vi "UI sbRIO9623.vi"(8 "error in":errorcluster) -> (0 "error out":errorcluster)   [LabVIEW 2019, in "sbRIO9623.lvlib"]
uses:
  sbRIO9623.lvlib
  SubVI/IO Control.ctl
  SubVI/LED Indicator.ctl
  User Event/Controls/UE Abort Action.ctl
  <vilib>/Utility/miscctls.llb/LVPointTypeDef.ctl
  <vilib>/Utility/error.llb/Error Cluster From Error Code.vi
  <vilib>/FPGAPlugInAG/sbRIO-9623/niLvFpga_Open_sbRIO-9623.vi
  <vilib>/rvi/interface/common/dynamic/niFpgaDynamicAddResources.vi
  <vilib>/FPGAPlugInAG/Dynamic/niLvFpga_Reset_Dynamic.vi
  <vilib>/FPGAPlugInAG/Dynamic/niLvFpga_Run_Dynamic.vi
  <vilib>/rvi/errors/niLvFpgaAdjustHostInterfaceError.vi
  <vilib>/rvi/interface/common/niFpgaWaitOnOcc.vi
  <vilib>/FPGAPlugInAG/Dynamic/niLvFpga_Close_Dynamic.vi
  <vilib>/ErrorRing/Error Ring.xnode
  <vilib>/rvi/interface/nirviOpenFPGA/nirviOpenFPGA.xnode
  SubVI/LabDevice_FPGATarget_FPGA0505A2015_bllO38D53-U.lvbitx
  <vilib>/rvi/interface/nirviMethod/nirviMethod.xnode
  <vilib>/rvi/interface/nirviReadWriteControl/nirviReadWriteControl.xnode
  <vilib>/rvi/interface/nirviCloseFPGA/nirviCloseFPGA.xnode
  Queues/Queues.lvlib
  NiFpgaLv.dll
  <vilib>/rvi/interface/Simulation/niFpgaSimulationCallBeginRW.vi
  <vilib>/FPGAPlugInAG/Dynamic/niLvFpga_ConfigureFifo_Dynamic.vi
  <vilib>/rvi/errors/niLvFpgaMergeErrorWithErrorCode.vi
panel:
  in  "LED Indicator":T1
  out "Sensor Indicator":T2
  out "SiPM 2":dbl(graph) caption="Waveform Chart - dark"
  out "SiPM 1":dbl(graph) caption="Waveform Chart - dark"
  in  "I/O Control":T3
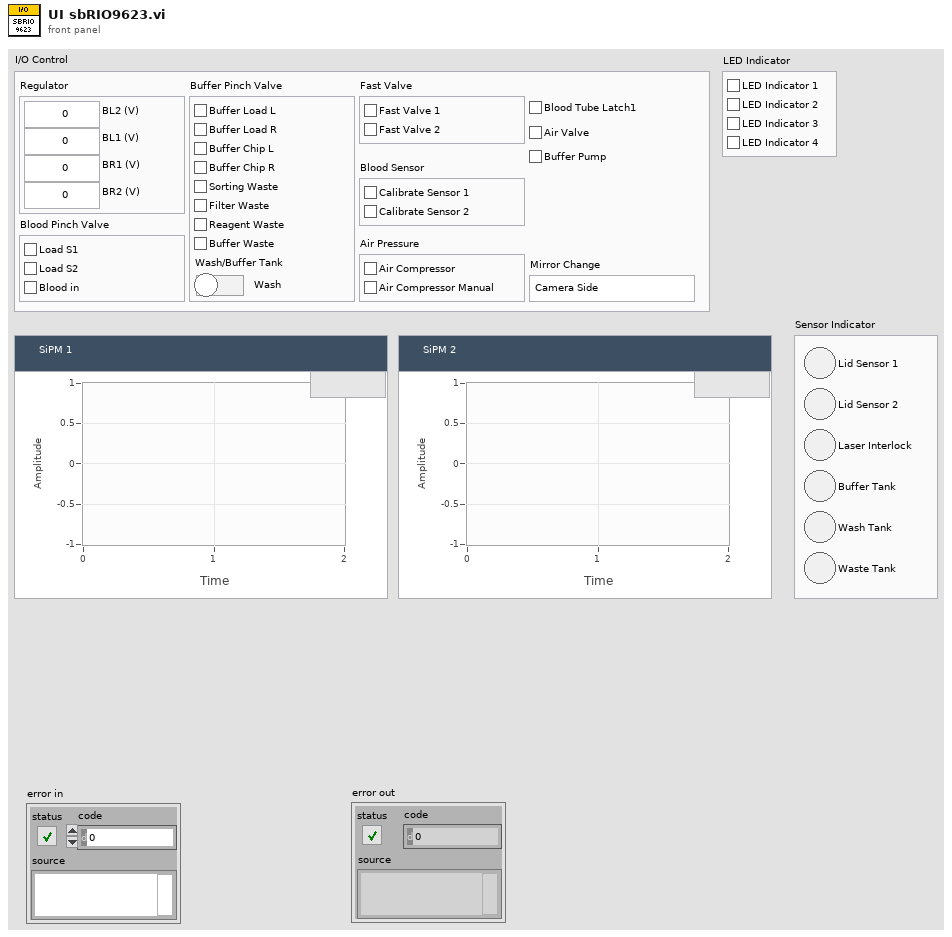
[diagram p1: front panel]
types:
  T1 = typedef "sbRIO9623.lvlib/LED Indicator.ctl" = cluster{"LED Indicator 1":bool, "LED Indicator 2":bool, "LED Indicator 3":bool, "LED Indicator 4":bool}
  T2 = cluster{"Lid Sensor 1":bool, "Lid Sensor 2":bool, "Laser Interlock":bool, "Buffer Tank":bool, "Wash Tank":bool, "Waste Tank":bool}
  T3 = typedef "sbRIO9623.lvlib/IO Control.ctl" = cluster{"Regulator":cluster{"BL2 (V)":fxp<+,16,3>, "BL1 (V)":fxp<+,16,3>, "BR1 (V)":fxp<+,16,3>, "BR2 (V)":fxp<+,16,3>}, "Buffer Pinch Valve":cluster{"Buffer Load L":bool, "Buffer Load R":bool, "Buffer Chip L":bool, "Buffer Chip R":bool, "Sorting Waste":bool, "Filter Waste":bool, "Reagent Waste":bool, "Buffer Waste":bool, "Wash/Buffer Tank":bool}, "Blood Pinch Valve":cluster{"Load S1":bool, "Load S2":bool, "Blood in":bool}, "Fast Valve":cluster{"Fast Valve 1":bool, "Fast Valve 2":bool}, "Blood Sensor":cluster{"Calibrate Sensor 1":bool, "Calibrate Sensor 2":bool}, "Air Pressure":cluster{"Air Compressor":bool, "Air Compressor Manual":bool}, "Blood Tube Latch1":bool, "Air Valve":bool, "Buffer Pump":bool, "Mirror Change":enum16{"Camera Side", "SiPM Side"}}
  T4 = cluster{"FPGA Ref":refnum<k20>, "Initialize Sucess?":bool, "Mirror Change":enum16{"Camera Side", "SiPM Side"}, "Air Pressure Control":cluster{"Air Compressor":bool, "Air Compressor (Manual)":bool, "Air Cmpressor Auto":bool}}
  T5 = typedef "UE Abort Action.ctl" = enum16{"Create", "Get", "Destroy"}
  T6 = cluster{"Wash Buffer Tank":bool, "Buffer Load L":bool, "Buffer Pump":bool}
  T7 = cluster{"Wash Buffer Tank":bool, "Buffer Load R":bool, "Buffer Pump":bool}
  T8 = cluster{"BR1":fxp<+,16,3>, "Buffer Chip R":bool, "Fast Valve 1":bool}
  T9 = cluster{"BR2":fxp<+,16,3>, "Buffer Chip R":bool, "Fast Valve 2":bool}
  T10 = typedef "LVPointTypeDef.ctl" = cluster{"Horizontal":i16, "Vertical":i16}
  T11 = typedef "sbRIO9623.lvlib/SEQ Data.ctl" = cluster{"Lid Sensor 1":bool, "Lid Sensor 2":bool, "Laser Interlock":bool, "Buffer Tank":bool, "Wash Tank":bool, "Waste Tank":bool, "SiPM 1":fxp<+,20,5>, "SiPM 2":fxp<+,20,5>, "Initialize Success?":bool, "VI Refnum":refnum<vi>}
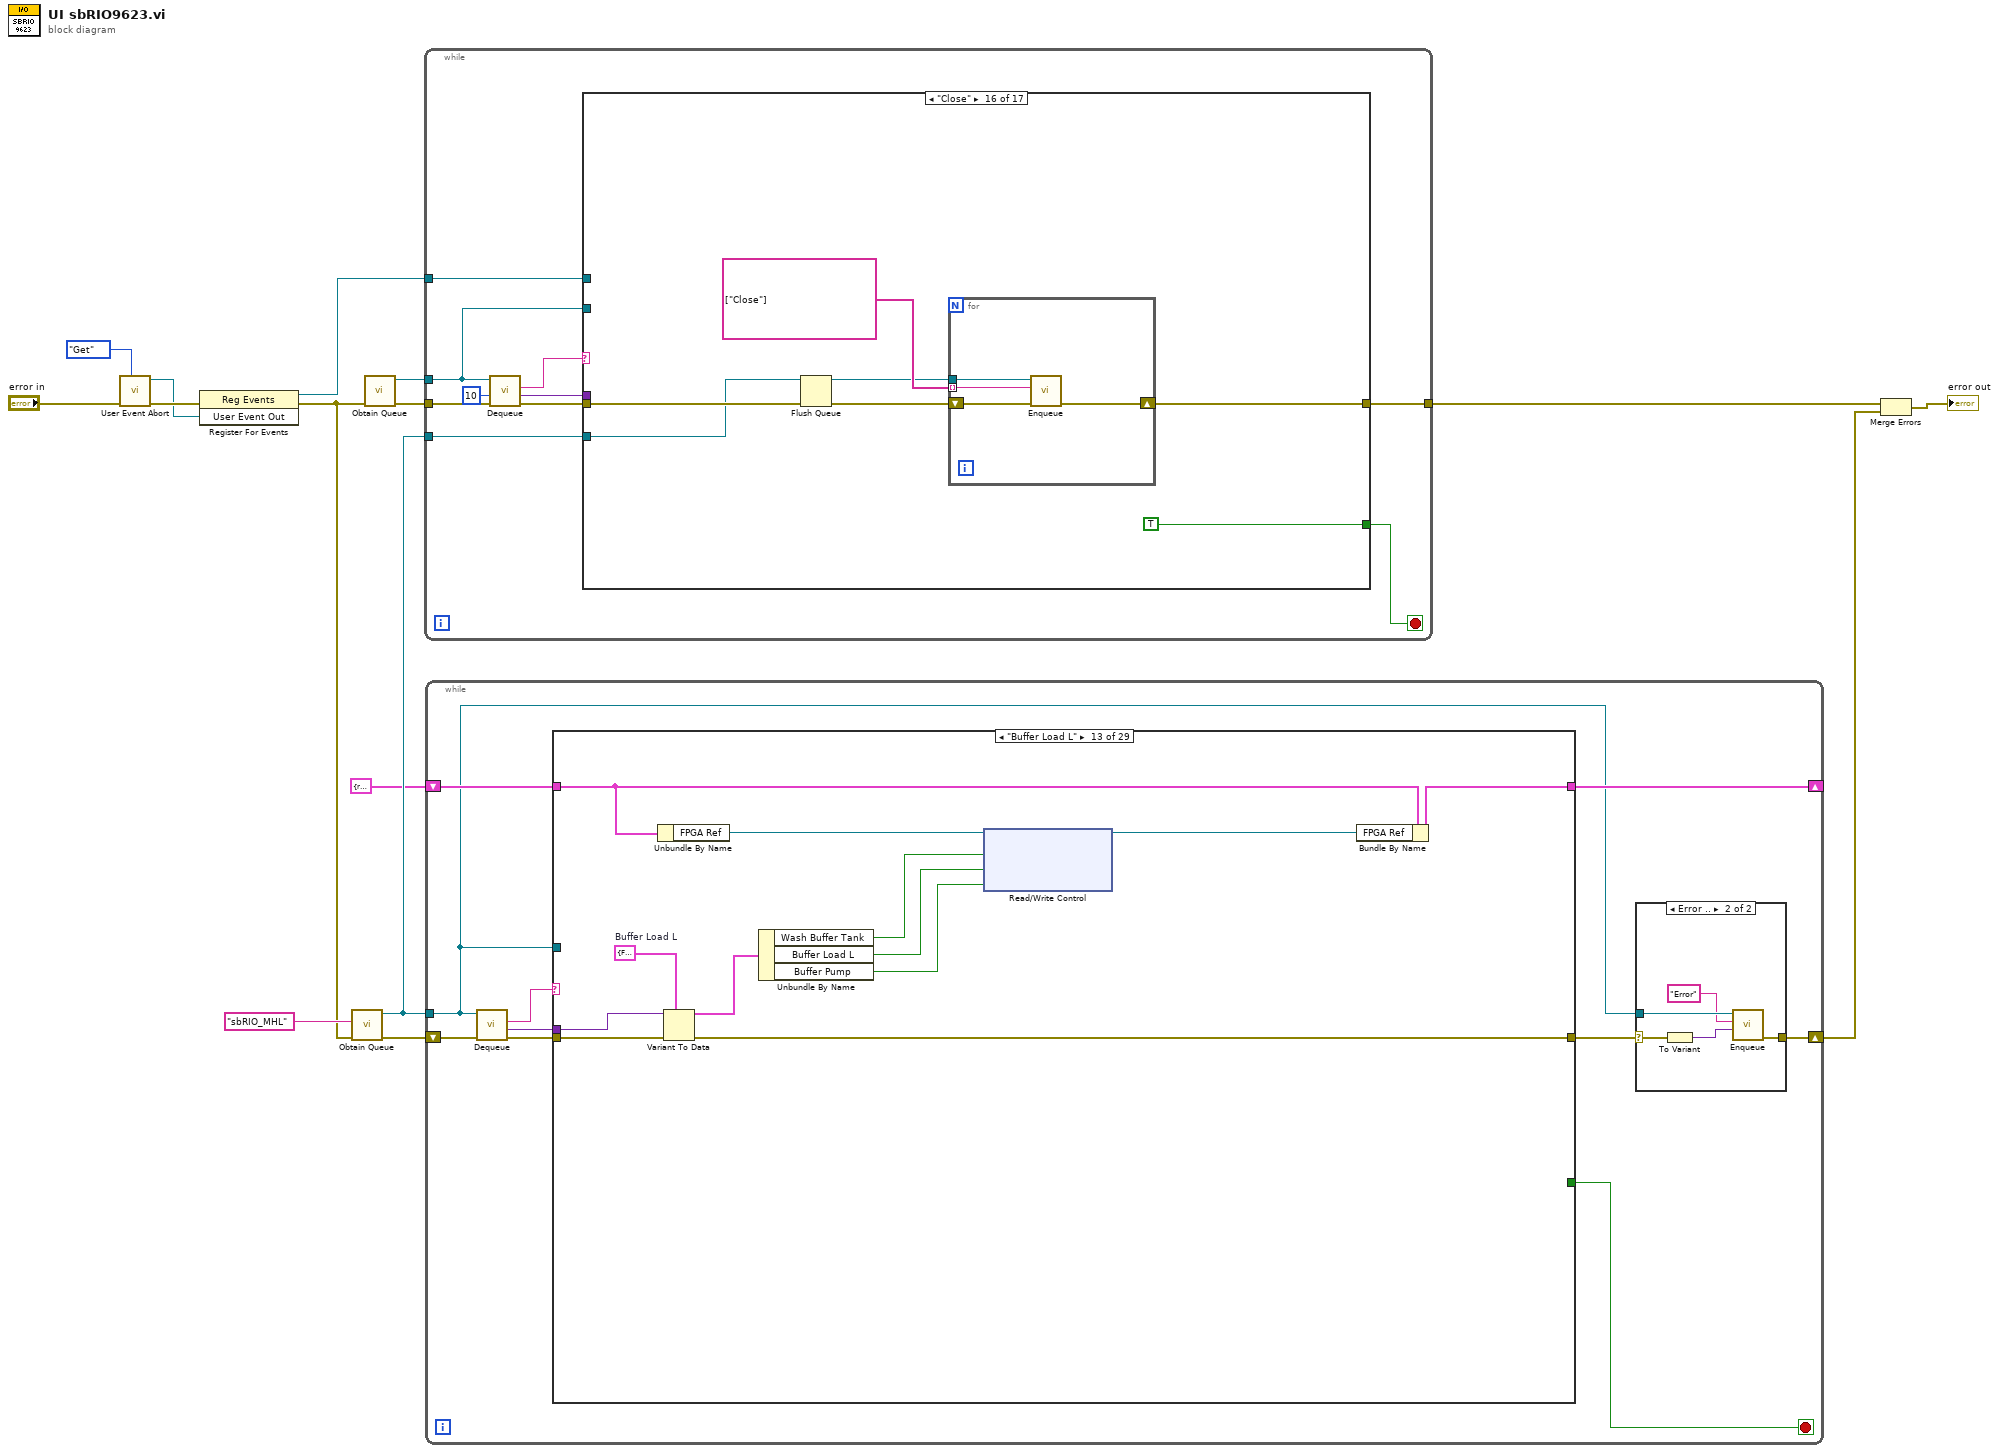
[diagram p0: block diagram]
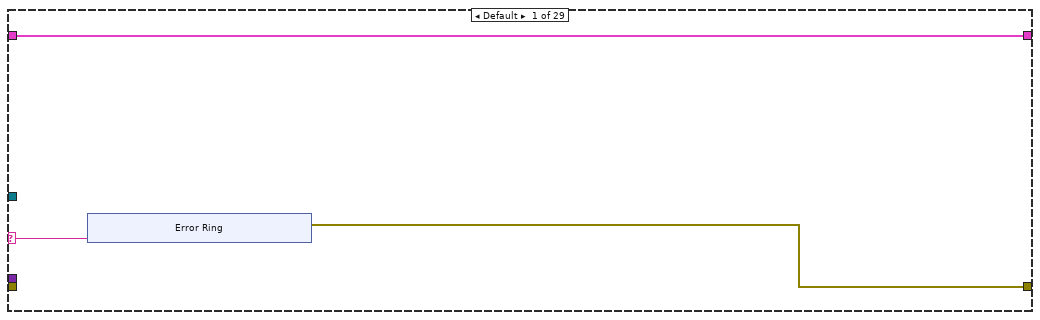
[diagram p2: hidden frame]
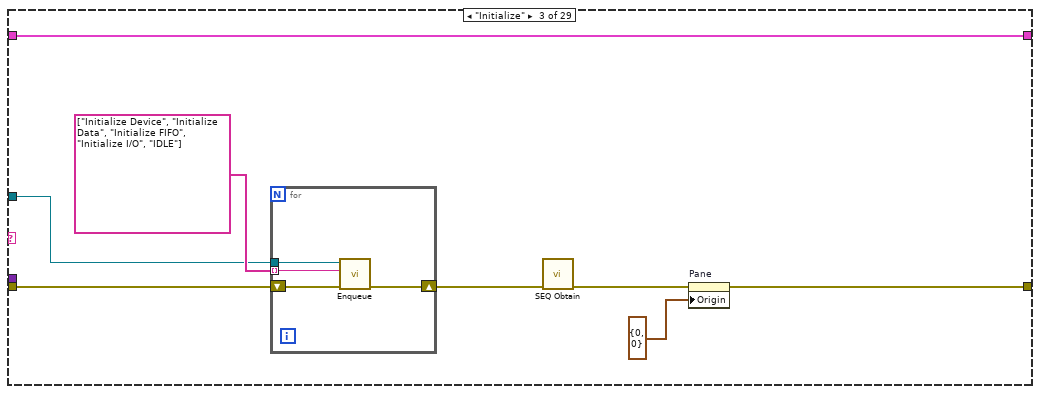
[diagram p4: hidden frame]
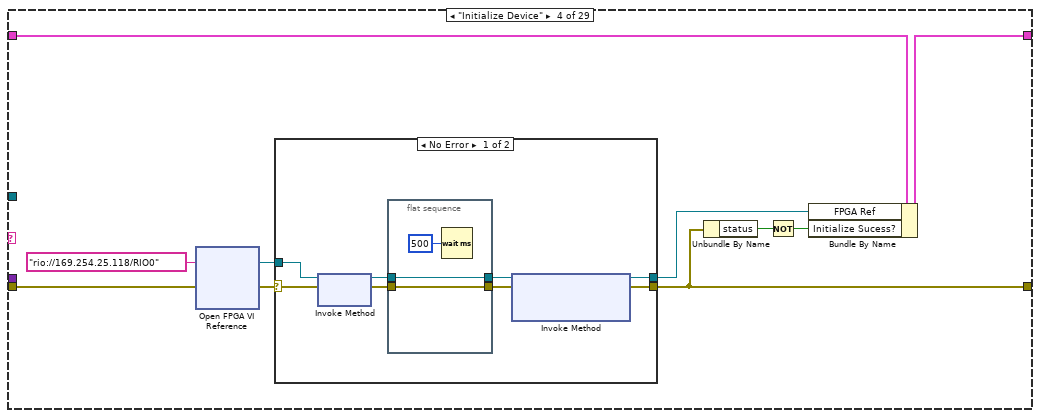
[diagram p5: hidden frame]
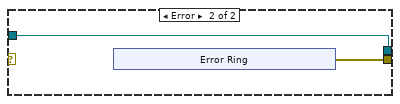
[diagram p6: hidden frame]
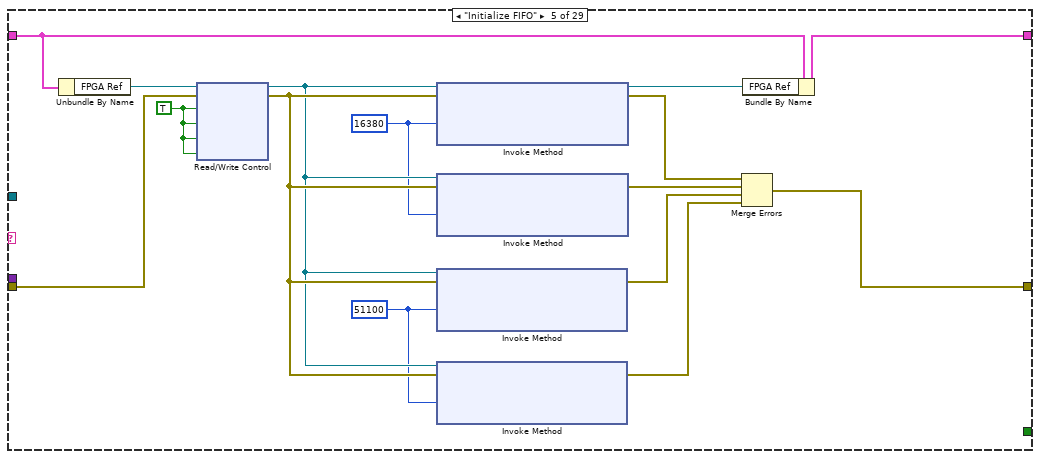
[diagram p7: hidden frame]
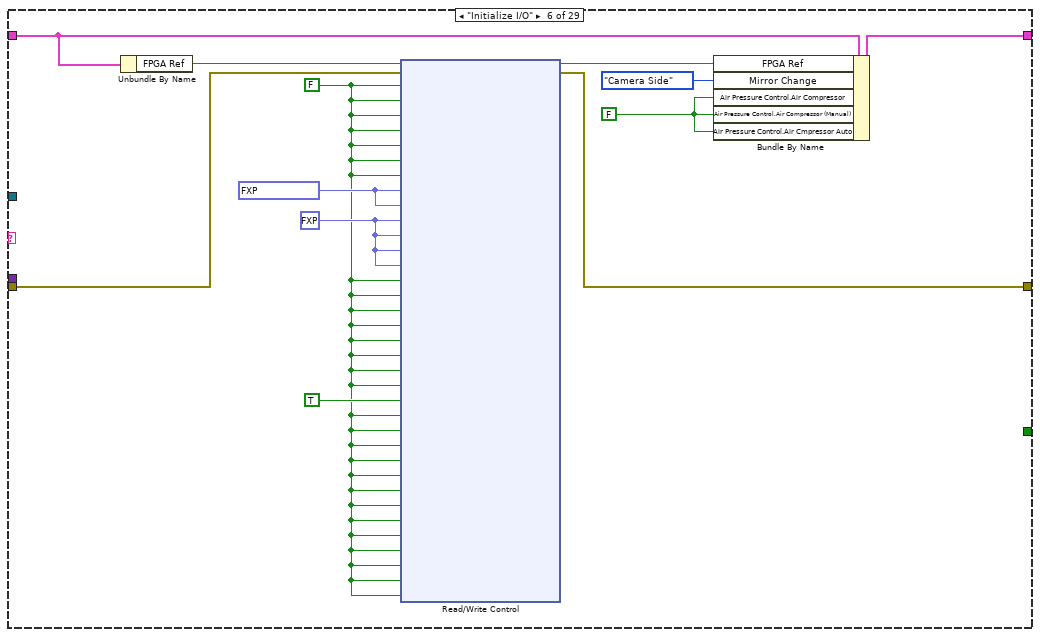
[diagram p8: hidden frame]
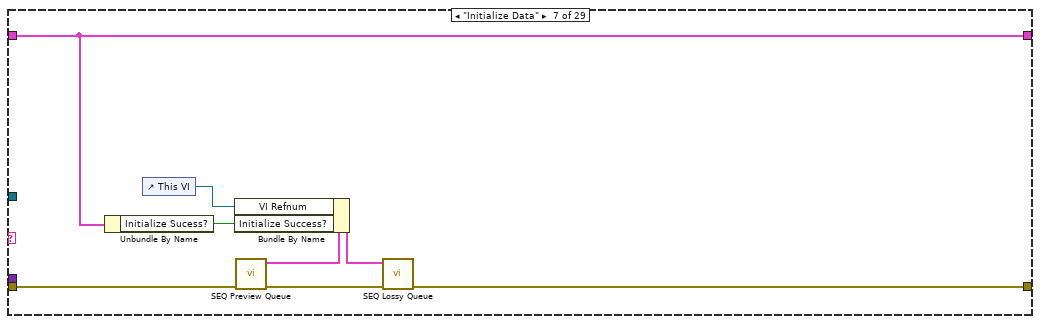
[diagram p9: hidden frame]
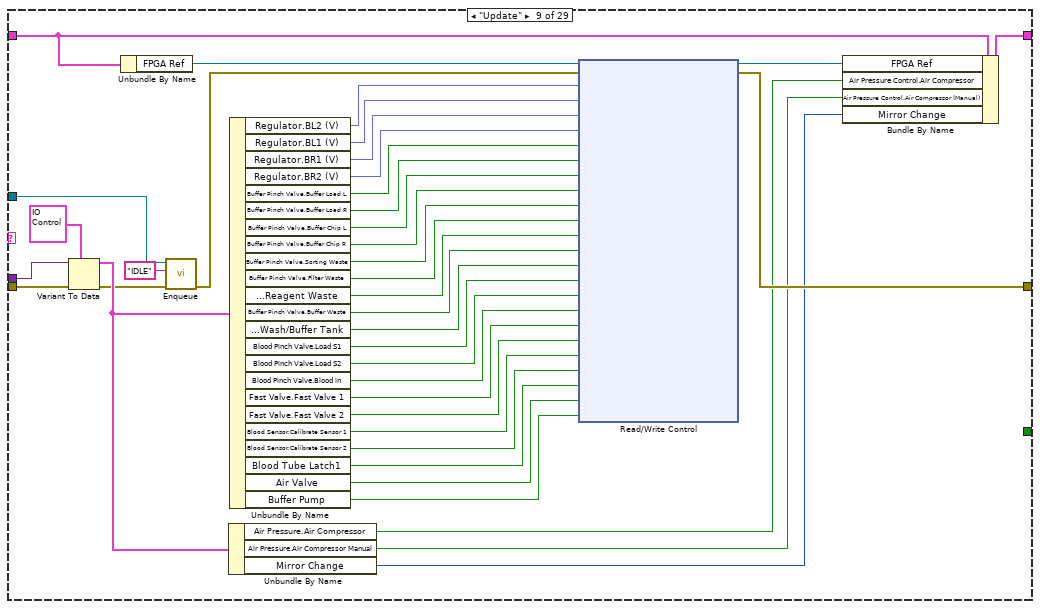
[diagram p11: hidden frame]
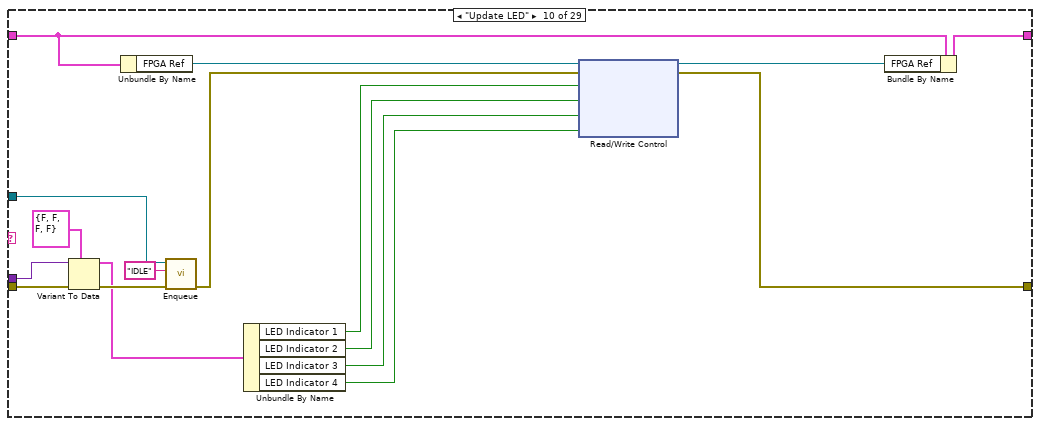
[diagram p12: hidden frame]
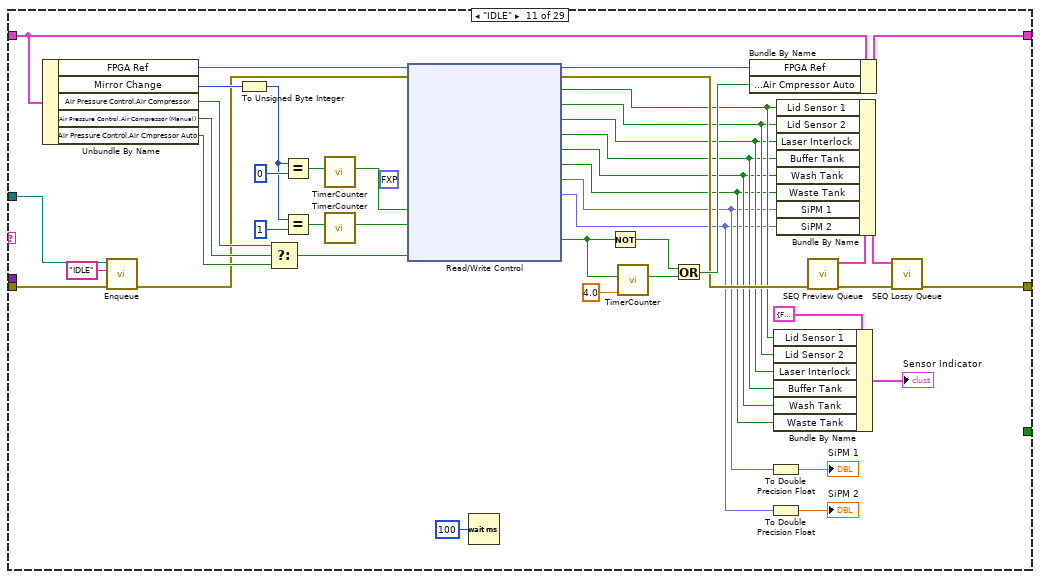
[diagram p13: hidden frame]
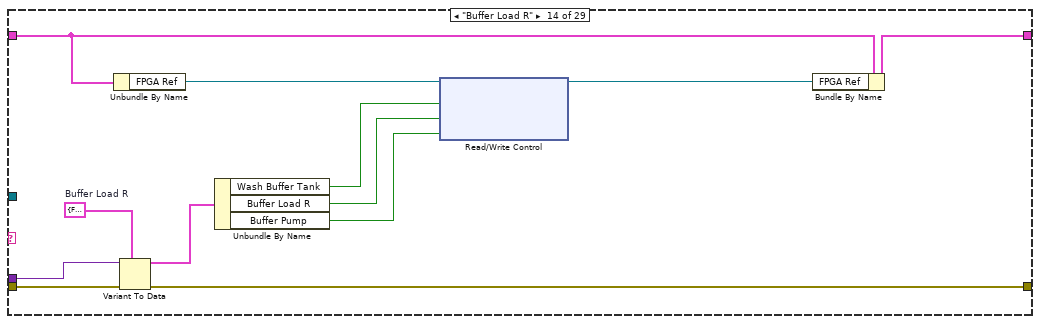
[diagram p15: hidden frame]
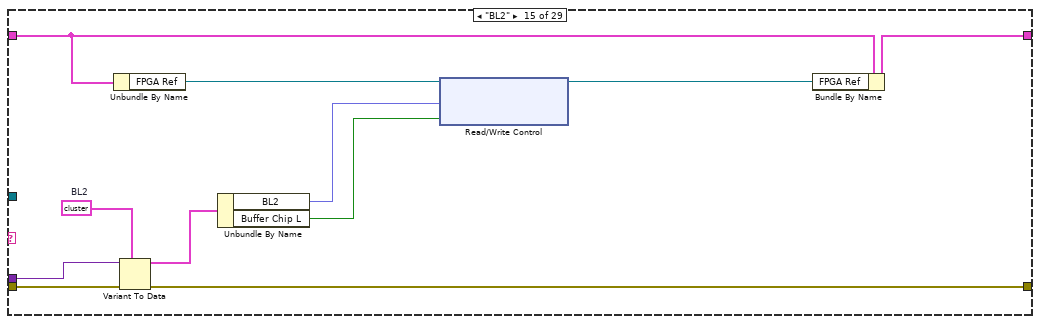
[diagram p16: hidden frame]
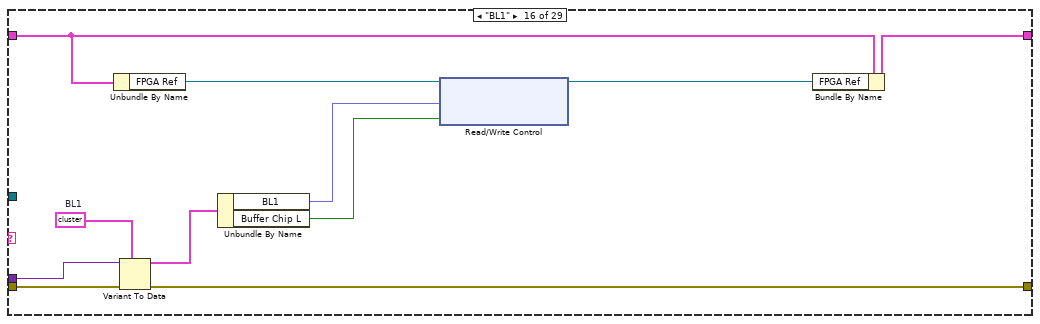
[diagram p17: hidden frame]
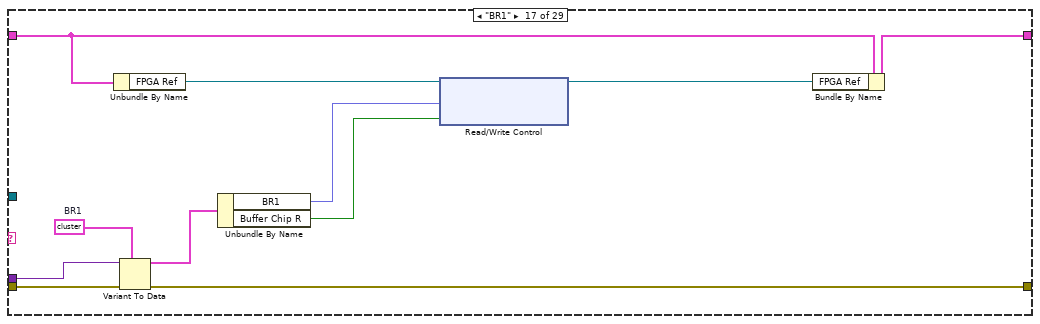
[diagram p18: hidden frame]
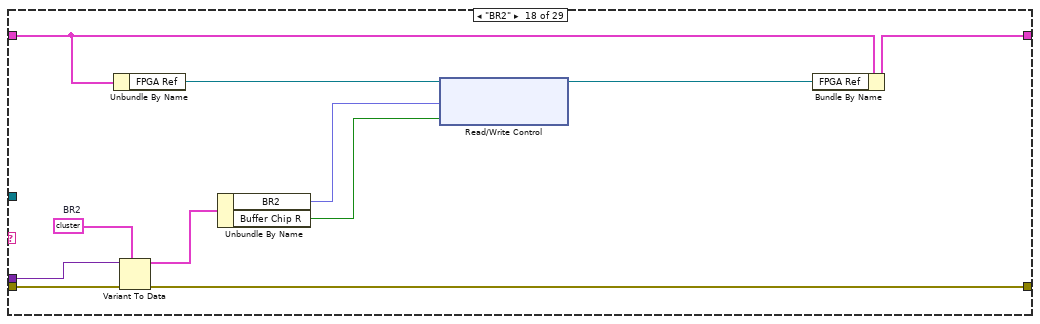
[diagram p19: hidden frame]
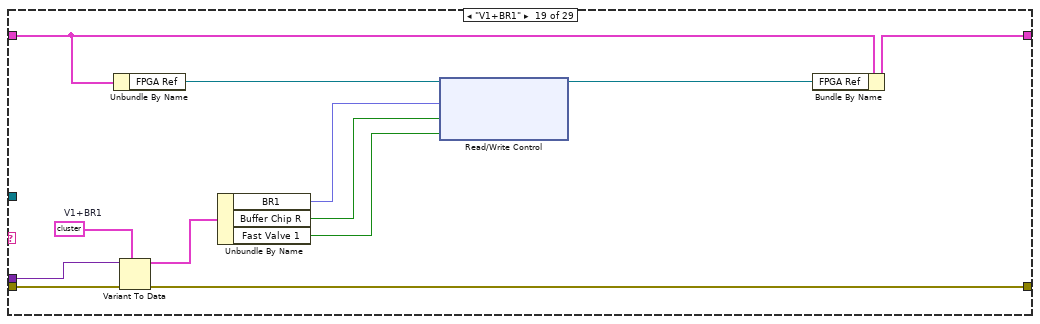
[diagram p20: hidden frame]
diagram:
  n1 = call "User Event Abort.vi"("Action"=UE_Abort_Action."Get", "Error In"="error in") -> ("Error Out"=w13:errorcluster, "User Event Out"=w12:refnum<user-event>)  [unwired: 8 in]
  n2 = register-events(error in=w13, w12) -> (reference out=w11:refnum<event-registration>, error out=w3:errorcluster)  [unwired: 1 in]
  n3 = call "Obtain Queue.vi"("Error In"=w3, "Queue Name"="sbRIO_MHL") -> ("Error Out"=w9:errorcluster, "queue out"=w5:refnum<queue>)  [unwired: 8 in]
  n4 = call "Obtain Queue.vi"("Error In"=w3) -> ("Error Out"=w2:errorcluster, "Queue out"=w1:refnum<queue>)  [unwired: 9 in]
  n5 = while {
    tunnel: w2 -> [w25]
    tunnel: w1 -> [w20]
    tunnel: [w19] -> w8
    tunnel: w11 -> [w18]
    tunnel: w5 -> [w16]
    stop <- w17 stop-if-true
    n6 = call "Dequeue.vi"("Error In"=w25, "timeout in ms (-1)"=10, "Queue in"=w20) -> ("Error Out"=w24:errorcluster, "Data"=w22:variant, "State"=w23:string)  [unwired: 5 in, 1 out]
    n7 = case shown="\"Close\"" w23 {
      selector: w23 -> [w26 _ _ _ _ _ _ _ _ _ _ _ _ _ _ _ _]
      tunnel: w24 -> [w29 w33 w46 w57 w67 w79 w91 w103 w115 w127 w139 w151 w163 w175 w187 w195 w206]
      tunnel: w22 -> [_ _ w45 w56 w66 w78 w90 w102 w114 w126 w138 w150 w162 w174 w186 _ _]
      tunnel: w20 -> [_ _ _ _ _ _ _ _ _ _ _ _ _ _ _ _ _]
      tunnel: [w29 w32 w42 w54 w65 w77 w89 w101 w113 w125 w137 w149 w161 w173 w185 w197 w205] -> w19
      tunnel: w18 -> [_ _ _ _ _ _ _ _ _ _ _ _ _ _ _ _ w204]
      tunnel: [_ _ _ _ _ _ _ _ _ _ _ _ _ _ _ TRUE _] -> w17
      tunnel: w16 -> [_ w31 w39 w50 w63 w75 w87 w99 w111 w123 w135 w147 w159 w171 w183 w192 w203]
      frame "Typo", Default {
        n8 = Concatenate Strings("Typo: " ("string"), w26) -> (w28:string)
        n9 = One Button Dialog(message=w28) -> ()  [unwired: 1 in, 1 out]
      }
      frame "Initialize" {
        n10 = for {
          tunnel: w31 -> [w35]
          shift-right: [w36] -> w32
          shift-left: w33 -> [w37]
          tunnel: string[] ["Initialize"] -> [w34] mode=indexing
          n11 = call "Enqueue.vi"("Error In"=w37, "State"=w34, "Queue in"=w35) -> ("Error Out"=w36:errorcluster)  [unwired: 7 in, 1 out]
        }
      }
      frame "Update" {
        n12 = Variant To Data(error in=w46, type=T3 {"Regulator"={"BL2 (V)"=0.0, "BL1 (V)"=0.0, "BR1 (V)"=0.0, "BR2 (V)"=0.0}, "Buffer Pinch Valve"={"Buffer Load L"=FALSE, "Buffer Load R"=FALSE, "Buffer Chip L"=FALSE, "Buffer Chip R"=FALSE, "Sorting Waste"=FALSE, "Filter Waste"=FALSE, "Reagent Waste"=FALSE, "Buffer Waste"=FALSE, "Wash/Buffer Tank"=FALSE}, "Blood Pinch Valve"={"Load S1"=FALSE, "Load S2"=FALSE, "Blood in"=FALSE}, "Fast Valve"={"Fast Valve 1"=FALSE, "Fast Valve 2"=FALSE}, "Blood Sensor"={"Calibrate Sensor 1"=FALSE, "Calibrate Sensor 2"=FALSE}, "Air Pressure"={"Air Compressor"=FALSE, "Air Compressor Manual"=FALSE}, "Blood Tube Latch1"=FALSE, "Air Valve"=FALSE, "Buffer Pump"=FALSE, "Mirror Change"=enum."Camera Side"} ("I/O Control"), Variant=w45) -> (data=w43:T3, error out=w41:errorcluster)
        n13 = To Variant(anything=w43) -> (Variant=w48:variant)
        n14 = Flush Queue(queue=w39, error in (no error)=w41) -> (queue out=w38:refnum<queue>, error out=w40:errorcluster)  [unwired: 1 out]
        n15 = call "Enqueue.vi"("Error In"=w40, "Data"=w48, "State"="Update", "Queue in"=w38) -> ("Error Out"=w42:errorcluster)  [unwired: 6 in, 1 out]
      }
      frame "Update LED" {
        n16 = Variant To Data(error in=w57, type=T1 {"LED Indicator 1"=FALSE, "LED Indicator 2"=FALSE, "LED Indicator 3"=FALSE, "LED Indicator 4"=FALSE} ("LED Indicator"), Variant=w56) -> (data=w55:T1, error out=w52:errorcluster)
        n17 = To Variant(anything=w55) -> (Variant=w59:variant)
        n18 = Flush Queue(queue=w50, error in (no error)=w52) -> (queue out=w49:refnum<queue>, error out=w51:errorcluster)  [unwired: 1 out]
        n19 = call "Enqueue.vi"("Error In"=w51, "Data"=w59, "State"="Update LED", "Queue in"=w49) -> ("Error Out"=w54:errorcluster)  [unwired: 6 in, 1 out]
      }
      frame "Buffer Load L" {
        n20 = Variant To Data(error in=w67, type=FALSE, Variant=w66) -> (data=w61:bool, error out=w62:errorcluster)
        n21 = case shown="True" w61 {
          tunnel: [w70 w71] -> w60
          frame True {
            w70 = T6 {"Wash Buffer Tank"=TRUE, "Buffer Load L"=TRUE, "Buffer Pump"=TRUE}  # Buffer Load L
          }
          frame False {
            w71 = T6 {"Wash Buffer Tank"=FALSE, "Buffer Load L"=FALSE, "Buffer Pump"=FALSE}  # Buffer Load L
          }
        }
        n22 = To Variant(anything=w60) -> (Variant=w69:variant)
        n23 = call "Enqueue.vi"("Error In"=w62, "Data"=w69, "State"="Buffer Load L", "Queue in"=w63) -> ("Error Out"=w65:errorcluster)  [unwired: 6 in, 1 out]
      }
      frame "Buffer Load R" {
        n24 = Variant To Data(error in=w79, type=FALSE, Variant=w78) -> (data=w73:bool, error out=w74:errorcluster)
        n25 = case shown="True" w73 {
          tunnel: [w82 w83] -> w72
          frame True {
            w82 = T7 {"Wash Buffer Tank"=TRUE, "Buffer Load R"=TRUE, "Buffer Pump"=TRUE}  # Buffer Load R
          }
          frame False {
            w83 = T7 {"Wash Buffer Tank"=FALSE, "Buffer Load R"=FALSE, "Buffer Pump"=FALSE}  # Buffer Load R
          }
        }
        n26 = To Variant(anything=w72) -> (Variant=w81:variant)
        n27 = call "Enqueue.vi"("Error In"=w74, "Data"=w81, "State"="Buffer Load R", "Queue in"=w75) -> ("Error Out"=w77:errorcluster)  [unwired: 6 in, 1 out]
      }
      frame "BL2" {
        n28 = Variant To Data(error in=w91, type=FALSE, Variant=w90) -> (data=w85:bool, error out=w86:errorcluster)
        n29 = case shown="True" w85 {
          tunnel: [w94 w95] -> w84
          frame True {
            w94 = cluster{"BL2":fxp<+,16,3>, "Buffer Chip L":bool} {"BL2"=0.5, "Buffer Chip L"=TRUE}  # BL2
          }
          frame False {
            w95 = cluster{"BL2":fxp<+,16,3>, "Buffer Chip L":bool} {"BL2"=0.0, "Buffer Chip L"=FALSE}  # BL2
          }
        }
        n30 = To Variant(anything=w84) -> (Variant=w93:variant)
        n31 = call "Enqueue.vi"("Error In"=w86, "Data"=w93, "State"="BL2", "Queue in"=w87) -> ("Error Out"=w89:errorcluster)  [unwired: 6 in, 1 out]
      }
      frame "BL1" {
        n32 = Variant To Data(error in=w103, type=FALSE, Variant=w102) -> (data=w97:bool, error out=w98:errorcluster)
        n33 = case shown="True" w97 {
          tunnel: [w106 w107] -> w96
          frame True {
            w106 = cluster{"BL1":fxp<+,16,3>, "Buffer Chip L":bool} {"BL1"=0.5, "Buffer Chip L"=TRUE}  # BL1
          }
          frame False {
            w107 = cluster{"BL1":fxp<+,16,3>, "Buffer Chip L":bool} {"BL1"=0.0, "Buffer Chip L"=FALSE}  # BL1
          }
        }
        n34 = To Variant(anything=w96) -> (Variant=w105:variant)
        n35 = call "Enqueue.vi"("Error In"=w98, "Data"=w105, "State"="BL1", "Queue in"=w99) -> ("Error Out"=w101:errorcluster)  [unwired: 6 in, 1 out]
      }
      frame "BR1" {
        n36 = Variant To Data(error in=w115, type=FALSE, Variant=w114) -> (data=w109:bool, error out=w110:errorcluster)
        n37 = case shown="True" w109 {
          tunnel: [w118 w119] -> w108
          frame True {
            w118 = cluster{"BR1":fxp<+,16,3>, "Buffer Chip R":bool} {"BR1"=0.5, "Buffer Chip R"=TRUE}  # BR1
          }
          frame False {
            w119 = cluster{"BR1":fxp<+,16,3>, "Buffer Chip R":bool} {"BR1"=0.0, "Buffer Chip R"=FALSE}  # BR1
          }
        }
        n38 = To Variant(anything=w108) -> (Variant=w117:variant)
        n39 = call "Enqueue.vi"("Error In"=w110, "Data"=w117, "State"="BR1", "Queue in"=w111) -> ("Error Out"=w113:errorcluster)  [unwired: 6 in, 1 out]
      }
      frame "BR2" {
        n40 = Variant To Data(error in=w127, type=FALSE, Variant=w126) -> (data=w121:bool, error out=w122:errorcluster)
        n41 = case shown="True" w121 {
          tunnel: [w130 w131] -> w120
          frame True {
            w130 = cluster{"BR2":fxp<+,16,3>, "Buffer Chip R":bool} {"BR2"=0.5, "Buffer Chip R"=TRUE}  # BR2
          }
          frame False {
            w131 = cluster{"BR2":fxp<+,16,3>, "Buffer Chip R":bool} {"BR2"=0.0, "Buffer Chip R"=FALSE}  # BR2
          }
        }
        n42 = To Variant(anything=w120) -> (Variant=w129:variant)
        n43 = call "Enqueue.vi"("Error In"=w122, "Data"=w129, "State"="BR2", "Queue in"=w123) -> ("Error Out"=w125:errorcluster)  [unwired: 6 in, 1 out]
      }
      frame "V1+BR1" {
        n44 = Variant To Data(error in=w139, type=FALSE, Variant=w138) -> (data=w133:bool, error out=w134:errorcluster)
        n45 = case shown="True" w133 {
          tunnel: [w142 w143] -> w132
          frame True {
            w142 = T8 {"BR1"=0.5, "Buffer Chip R"=TRUE, "Fast Valve 1"=TRUE}  # V1+BR1
          }
          frame False {
            w143 = T8 {"BR1"=0.0, "Buffer Chip R"=FALSE, "Fast Valve 1"=FALSE}  # V1+BR1
          }
        }
        n46 = To Variant(anything=w132) -> (Variant=w141:variant)
        n47 = call "Enqueue.vi"("Error In"=w134, "Data"=w141, "State"="V1+BR1", "Queue in"=w135) -> ("Error Out"=w137:errorcluster)  [unwired: 6 in, 1 out]
      }
      frame "V2+BR2" {
        n48 = Variant To Data(error in=w151, type=FALSE, Variant=w150) -> (data=w145:bool, error out=w146:errorcluster)
        n49 = case shown="True" w145 {
          tunnel: [w154 w155] -> w144
          frame True {
            w154 = T9 {"BR2"=0.5, "Buffer Chip R"=TRUE, "Fast Valve 2"=TRUE}  # V2+BR2
          }
          frame False {
            w155 = T9 {"BR2"=0.0, "Buffer Chip R"=FALSE, "Fast Valve 2"=FALSE}  # V2+BR2
          }
        }
        n50 = To Variant(anything=w144) -> (Variant=w153:variant)
        n51 = call "Enqueue.vi"("Error In"=w146, "Data"=w153, "State"="V2+BR2", "Queue in"=w147) -> ("Error Out"=w149:errorcluster)  [unwired: 6 in, 1 out]
      }
      frame "REA" {
        n52 = Variant To Data(error in=w163, type=FALSE, Variant=w162) -> (data=w157:bool, error out=w158:errorcluster)
        n53 = case shown="True" w157 {
          tunnel: [w166 w167] -> w156
          frame True {
            w166 = cluster{"BL2":fxp<+,16,3>, "Air Valve":bool} {"BL2"=0.5, "Air Valve"=TRUE}  # REA
          }
          frame False {
            w167 = cluster{"BL2":fxp<+,16,3>, "Air Valve":bool} {"BL2"=0.0, "Air Valve"=FALSE}  # REA
          }
        }
        n54 = To Variant(anything=w156) -> (Variant=w165:variant)
        n55 = call "Enqueue.vi"("Error In"=w158, "Data"=w165, "State"="REA", "Queue in"=w159) -> ("Error Out"=w161:errorcluster)  [unwired: 6 in, 1 out]
      }
      frame "SW1/2" {
        n56 = Variant To Data(error in=w175, type=FALSE, Variant=w174) -> (data=w169:bool, error out=w170:errorcluster)
        n57 = case shown="True" w169 {
          tunnel: [w178 w179] -> w168
          frame True {
            w178 = cluster{"Sorting Waste":bool} {"Sorting Waste"=TRUE}  # SW1/2
          }
          frame False {
            w179 = cluster{"Sorting Waste":bool} {"Sorting Waste"=FALSE}  # SW1/2
          }
        }
        n58 = To Variant(anything=w168) -> (Variant=w177:variant)
        n59 = call "Enqueue.vi"("Error In"=w170, "Data"=w177, "State"="SW1/2", "Queue in"=w171) -> ("Error Out"=w173:errorcluster)  [unwired: 6 in, 1 out]
      }
      frame "FW1/2" {
        n60 = Variant To Data(error in=w187, type=FALSE, Variant=w186) -> (data=w181:bool, error out=w182:errorcluster)
        n61 = case shown="True" w181 {
          tunnel: [w190 w191] -> w180
          frame True {
            w190 = cluster{"Filter Waste":bool} {"Filter Waste"=TRUE}  # FW1/2
          }
          frame False {
            w191 = cluster{"Filter Waste":bool} {"Filter Waste"=FALSE}  # FW1/2
          }
        }
        n62 = To Variant(anything=w180) -> (Variant=w189:variant)
        n63 = call "Enqueue.vi"("Error In"=w182, "Data"=w189, "State"="FW1/2", "Queue in"=w183) -> ("Error Out"=w185:errorcluster)  [unwired: 6 in, 1 out]
      }
      frame "Close" {
        n64 = Flush Queue(queue=w192, error in (no error)=w195) -> (queue out=w193:refnum<queue>, error out=w194:errorcluster)  [unwired: 1 out]
        n65 = for {
          tunnel: w193 -> [w200]
          shift-right: [w201] -> w197
          shift-left: w194 -> [w202]
          tunnel: string[] ["Close"] -> [w199] mode=indexing
          n66 = call "Enqueue.vi"("Error In"=w202, "State"=w199, "Queue in"=w200) -> ("Error Out"=w201:errorcluster)  [unwired: 7 in, 1 out]
        }
      }
      frame "Idle" {
        n67 = event shown="[0] Timeout" {
          selector: w204 -> [_ _ _ w218]
          dyn-events: _ -> [_ _ _ _]
          timeout: 10 -> [_ _ _ _]
          tunnel: w206 -> [w208 w211 w213 w216]
          tunnel: [w208 w210 w212 w217] -> w205
          tunnel: w203 -> [_ _ _ _]
          event Timeout {
            n68 = event-data() -> ()  [unwired: 1 in, 3 out]
          }
          event Value Change {
            n69 = event-data() -> ()  [unwired: 1 in, 6 out]
            n70 = call "Update.vi"("Error In"=w211, "I/O Control"="I/O Control") -> ("Error Out"=w210:errorcluster)  [unwired: 9 in]
          }
          event Value Change {
            n71 = event-data() -> ()  [unwired: 1 in, 6 out]
            n72 = call "Update LED.vi"("Error In"=w213, "LED Indicator"="LED Indicator") -> ("Error Out"=w212:errorcluster)  [unwired: 9 in]
          }
          event User Event {
            n73 = event-data() -> ()  [unwired: 1 in, 4 out]
            n74 = call "Close.vi"("Error In"=w216) -> ("Error Out"=w215:errorcluster)  [unwired: 10 in]
            n75 = Unregister For Events(event registration refnum=w218, error in=w215) -> (error out=w217:errorcluster)
          }
        }
      }
    }
  }
  n76 = while {
    tunnel: w5 -> [w220]
    shift-right: [w223] -> _
    shift-left: T4 {"FPGA Ref"=refnum, "Initialize Sucess?"=FALSE, "Mirror Change"=enum."Camera Side", "Air Pressure Control"={"Air Compressor"=FALSE, "Air Compressor (Manual)"=FALSE, "Air Cmpressor Auto"=FALSE}} -> [w224]
    shift-right: [w222] -> w6
    shift-left: w9 -> [w228]
    stop <- w219 stop-if-true
    n77 = call "Dequeue.vi"("Error In"=w228, "Queue in"=w220) -> ("Error Out"=w225:errorcluster, "Data"=w226:variant, "State"=w227:string)  [unwired: 6 in, 1 out]
    n78 = case shown="\"Buffer Load L\"" w227 {
      selector: w227 -> [w230 _ _ _ _ _ _ _ _ _ _ _ _ _ _ _ _ _ _ _ _ _ _ _ _ _ _ _ _]
      tunnel: w220 -> [_ _ w246 _ _ _ _ _ w319 w364 w375 _ _ _ _ _ _ _ _ _ _ _ _ _ _ _ w554 _ w568]
      tunnel: w226 -> [_ _ _ _ _ _ _ _ w353 w370 _ _ w429 w441 w452 w463 w474 w485 w497 w509 w520 w530 w540 _ w546 _ _ _ _]
      tunnel: w225 -> [_ w239 w247 w262 w293 w301 w315 w317 w354 w371 w377 w417 w430 w442 w453 w464 w475 w486 w498 w510 w521 w531 w541 w543 w547 w551 w555 w564 w569]
      tunnel: w224 -> [w231 w240 w245 w258 w295 w307 w310 w316 w356 w373 w416 w418 w428 w440 w451 w462 w473 w484 w496 w508 w519 w529 w539 w542 w544 w550 w552 w563 w567]
      tunnel: [w231 w240 w245 w257 w285 w305 w310 w316 w355 w372 w414 w418 w427 w439 w450 w461 w472 w483 w495 w507 w518 w528 w538 w542 w544 w550 w552 w563 w567] -> w223
      tunnel: [w229 w239 w242 w255 w286 w299 w313 w317 w349 w367 w392 w417 w424 w436 w446 w457 w468 w479 w491 w503 w514 w524 w534 w543 errorcluster {"status"=FALSE, "code"=0, "source"=""} ("Error Out") w551 w553 w561 w565] -> w221
      tunnel: [_ _ _ _ _ _ _ _ _ _ _ _ _ _ _ _ _ _ _ _ _ _ _ _ _ _ _ _ TRUE] -> w219
      frame Default {
        n79 = xnode "Error Ring"("parameter 0"=w230) -> ("error out"=w229:errorcluster)
      }
      frame "------Initialize------" {
      }
      frame "Initialize" {
        n80 = for {
          tunnel: w246 -> [w250]
          shift-right: [w251] -> w244
          shift-left: w247 -> [w252]
          tunnel: string[] ["Initialize Device", "Initialize Data", "Initialize FIFO", "Initialize I/O", "IDLE"] -> [w249] mode=indexing
          n81 = call "Enqueue.vi"("Error In"=w252, "State"=w249, "Queue in"=w250) -> ("Error Out"=w251:errorcluster)  [unwired: 7 in, 1 out]
        }
        n82 = call "SEQ Obtain.vi"("error in"=w244) -> ("error out"=w243:errorcluster)  [unwired: 9 in, 1 out]
        n83 = property on="Pane" class="Pane"(error in=w243, "Origin"=T10 {"Horizontal"=0, "Vertical"=0}) -> (error out=w242:errorcluster)  [unwired: 1 in, 1 out]
      }
      frame "Initialize Device" {
        n84 = xnode "Open FPGA VI Reference"("error in"=w262, "resource name"=tag "rio://169.254.25.118/RIO0") -> ("FPGA VI Reference Out"=w260:refnum<k20>, "error out"=w259:errorcluster)
        n85 = case shown="No Error" w259 {
          selector: w259 -> [w269 _]
          tunnel: w260 -> [w270 w274]
          tunnel: [w264 w275] -> w255
          tunnel: [w263 w274] -> w256
          frame No Error {
            n86 = xnode "Invoke Method"("FPGA VI Reference In"=w270, "error in"=w269) -> ("FPGA VI Reference Out"=w267:refnum<k20>, "error out"=w268:errorcluster)
            n87 = flat-sequence {
              tunnel: w268 -> [w273]
              tunnel: [w273] -> w266
              tunnel: w267 -> [w272]
              tunnel: [w272] -> w265
              frame #0 {
                n88 = Wait (ms)(milliseconds to wait=u32 500) -> ()  [unwired: 1 out]
              }
            }
            n89 = xnode "Invoke Method"("FPGA VI Reference In"=w265, "error in"=w266) -> ("FPGA VI Reference Out"=w263:refnum<k20>, "error out"=w264:errorcluster)  [unwired: 1 in]
          }
          frame Error {
            n90 = xnode "Error Ring"() -> ("error out"=w275:errorcluster)
          }
        }
        n91 = Unbundle By Name(w255) -> ("status"=w254:bool)
        n92 = Not(x=w254) -> (.not. x?=w253:bool)
        n93 = Bundle By Name(cluster=w258, "FPGA Ref"=w256, "Initialize Sucess?"=w253) -> (w257:T4)
      }
      frame "Initialize FIFO" {
        w281 = u32 16380 ("Requested Depth")
        w282 = u32 51100 ("Requested Depth")
        w292 = TRUE ("LED Fan-1")
        n94 = Unbundle By Name(w295) -> ("FPGA Ref"=w294:refnum<k20>)
        n95 = xnode "Read/Write Control"("FPGA VI Reference In"=w294, "error in"=w293, "LED Fan-1"=w292, "LED Fan-2"=w292, "LED Fan-3"=w292, "LED Fan-4"=w292) -> ("FPGA VI Reference Out"=w284:refnum<k20>, "error out"=w291:errorcluster)
        n96 = xnode "Invoke Method"("FPGA VI Reference In"=w284, "error in"=w291, "Requested Depth"=w281) -> ("FPGA VI Reference Out"=w283:refnum<k20>, "error out"=w290:errorcluster)  [unwired: 1 out]
        n97 = xnode "Invoke Method"("FPGA VI Reference In"=w284, "error in"=w291, "Requested Depth"=w281) -> ("error out"=w289:errorcluster)  [unwired: 2 out]
        n98 = xnode "Invoke Method"("FPGA VI Reference In"=w284, "error in"=w291, "Requested Depth"=w282) -> ("error out"=w288:errorcluster)  [unwired: 2 out]
        n99 = xnode "Invoke Method"("FPGA VI Reference In"=w284, "error in"=w291, "Requested Depth"=w282) -> ("error out"=w287:errorcluster)  [unwired: 2 out]
        n100 = Merge Errors(w290, w289, w288, w287) -> (w286:errorcluster)
        n101 = Bundle By Name(cluster=w295, "FPGA Ref"=w283) -> (w285:T4)
      }
      frame "Initialize I/O" {
        w296 = FALSE ("Air Pressure Control.Air Compressor (Manual)")
        w303 = fxp<+,16,3> 0.0 ("regulatorcontrol2 (V)")
        w304 = fxp<+,20,5> 31.9990234375 ("TriggerLevel_sipm1")
        w298 = FALSE ("Baseline data?")
        n102 = Unbundle By Name(w307) -> ("FPGA Ref"=w306:refnum<k20>)
        n103 = xnode "Read/Write Control"("FPGA VI Reference In"=w306, "error in"=w301, "Baseline data?"=w298, "Air Compressor"=w298, "Indicator LED-1"=w298, "Indicator LED-2"=w298, "Indicator LED-3"=w298, "Indicator LED-4"=w298, "Buzzer Alarm"=w298, "TriggerLevel_sipm1"=w304, "TriggerLevel_sipm2"=w304, "regulatorcontrol2 (V)"=w303, "regulatorcontrol1 (V)"=w303, "regulatorcontrol3 (V)"=w303, "regulatorcontrol4 (V)"=w303, "Buffer Pinch Valve- 1"=w298, "Buffer Pinch Valve- 2"=w298, "Buffer Pinch Valve- 3"=w298, "Buffer Pinch Valve- 4"=w298, "Buffer Pinch Valve- 5"=w298, "Buffer Pinch Valve- 6"=w298, "Buffer Pinch Valve- 7"=w298, "Buffer Pinch Valve- 8"=w298, "Buffer Pinch Valve- 9"=TRUE, "Auto Fast Valve1"=w298, "Auto Fast Valve2"=w298, "FastValve1"=w298, "FastValve2"=w298, "Air Valve"=w298, "Blood Tube Latch-A"=w298, "Blood Tube Latch-B"=w298, "Buffer Pump"=w298, "Blood Sensor Calibration-1"=w298, "Blood Sensor Calibration-2"=w298, "Blood Pinch Valve-1"=w298, "Blood Pinch Valve-2"=w298, "Blood Pinch Valve-3"=w298) -> ("FPGA VI Reference Out"=w300:refnum<k20>, "error out"=w299:errorcluster)
        n104 = Bundle By Name(cluster=w307, "FPGA Ref"=w300, "Mirror Change"=enum16{"Camera Side", "SiPM Side"}."Camera Side", "Air Pressure Control.Air Compressor"=w296, "Air Pressure Control.Air Compressor (Manual)"=w296, "Air Pressure Control.Air Cmpressor Auto"=w296) -> (w305:T4)
      }
      frame "Initialize Data" {
        n105 = Unbundle By Name(w310) -> ("Initialize Sucess?"=w309:bool)
        n106 = control-ref of="This VI"() -> (w308:refnum<vi>)
        n107 = call "SEQ Preview Queue.vi"("error in"=w315) -> ("error out"=w314:errorcluster, "SEQ Data"=w312:T11)  [unwired: 9 in]
        n108 = Bundle By Name(cluster=w312, "VI Refnum"=w308, "Initialize Success?"=w309) -> (w311:T11)
        n109 = call "SEQ Lossy Queue.vi"("error in"=w314, "SEQ Data"=w311) -> ("error out"=w313:errorcluster)  [unwired: 9 in]
      }
      frame "------Functions------" {
      }
      frame "Update" {
        n110 = Variant To Data(error in=w354, type=T3 {"Regulator"={"BL2 (V)"=0.0, "BL1 (V)"=0.0, "BR1 (V)"=0.0, "BR2 (V)"=0.0}, "Buffer Pinch Valve"={"Buffer Load L"=FALSE, "Buffer Load R"=FALSE, "Buffer Chip L"=FALSE, "Buffer Chip R"=FALSE, "Sorting Waste"=FALSE, "Filter Waste"=FALSE, "Reagent Waste"=FALSE, "Buffer Waste"=FALSE, "Wash/Buffer Tank"=FALSE}, "Blood Pinch Valve"={"Load S1"=FALSE, "Load S2"=FALSE, "Blood in"=FALSE}, "Fast Valve"={"Fast Valve 1"=FALSE, "Fast Valve 2"=FALSE}, "Blood Sensor"={"Calibrate Sensor 1"=FALSE, "Calibrate Sensor 2"=FALSE}, "Air Pressure"={"Air Compressor"=FALSE, "Air Compressor Manual"=FALSE}, "Blood Tube Latch1"=FALSE, "Air Valve"=FALSE, "Buffer Pump"=FALSE, "Mirror Change"=enum."Camera Side"} ("I/O Control"), Variant=w353) -> (data=w325:T3, error out=w321:errorcluster)
        n111 = Unbundle By Name(w356) -> ("FPGA Ref"=w351:refnum<k20>)
        n112 = call "Enqueue.vi"("Error In"=w321, "State"="IDLE", "Queue in"=w319) -> ("Error Out"=w320:errorcluster)  [unwired: 7 in, 1 out]
        n113 = Unbundle By Name(w325) -> ("Air Pressure.Air Compressor"=w324:bool, "Air Pressure.Air Compressor Manual"=w323:bool, "Mirror Change"=w322:enum16{"Camera Side", "SiPM Side"})
        n114 = Unbundle By Name(w325) -> ("Regulator.BL2 (V)"=w348:fxp<+,16,3>, "Regulator.BL1 (V)"=w347:fxp<+,16,3>, "Regulator.BR1 (V)"=w346:fxp<+,16,3>, "Regulator.BR2 (V)"=w345:fxp<+,16,3>, "Buffer Pinch Valve.Buffer Load L"=w344:bool, "Buffer Pinch Valve.Buffer Load R"=w343:bool, "Buffer Pinch Valve.Buffer Chip L"=w342:bool, "Buffer Pinch Valve.Buffer Chip R"=w341:bool, "Buffer Pinch Valve.Sorting Waste"=w340:bool, "Buffer Pinch Valve.Filter Waste"=w339:bool, "Buffer Pinch Valve.Reagent Waste"=w338:bool, "Buffer Pinch Valve.Buffer Waste"=w337:bool, "Buffer Pinch Valve.Wash/Buffer Tank"=w336:bool, "Blood Pinch Valve.Load S1"=w335:bool, "Blood Pinch Valve.Load S2"=w334:bool, "Blood Pinch Valve.Blood in"=w333:bool, "Fast Valve.Fast Valve 1"=w332:bool, "Fast Valve.Fast Valve 2"=w331:bool, "Blood Sensor.Calibrate Sensor 1"=w330:bool, "Blood Sensor.Calibrate Sensor 2"=w329:bool, "Blood Tube Latch1"=w328:bool, "Air Valve"=w327:bool, "Buffer Pump"=w326:bool)
        n115 = xnode "Read/Write Control"("FPGA VI Reference In"=w351, "error in"=w320, "regulatorcontrol2 (V)"=w348, "regulatorcontrol1 (V)"=w347, "regulatorcontrol3 (V)"=w346, "regulatorcontrol4 (V)"=w345, "Buffer Pinch Valve- 1"=w344, "Buffer Pinch Valve- 2"=w343, "Buffer Pinch Valve- 3"=w342, "Buffer Pinch Valve- 4"=w341, "Buffer Pinch Valve- 5"=w340, "Buffer Pinch Valve- 6"=w339, "Buffer Pinch Valve- 7"=w338, "Buffer Pinch Valve- 8"=w337, "Buffer Pinch Valve- 9"=w336, "Blood Pinch Valve-1"=w335, "Blood Pinch Valve-2"=w334, "Blood Pinch Valve-3"=w333, "FastValve1"=w332, "FastValve2"=w331, "Blood Sensor Calibration-1"=w330, "Blood Sensor Calibration-2"=w329, "Blood Tube Latch-A"=w328, "Air Valve"=w327, "Buffer Pump"=w326) -> ("FPGA VI Reference Out"=w350:refnum<k20>, "error out"=w349:errorcluster)
        n116 = Bundle By Name(cluster=w356, "FPGA Ref"=w350, "Air Pressure Control.Air Compressor"=w324, "Air Pressure Control.Air Compressor (Manual)"=w323, "Mirror Change"=w322) -> (w355:T4)
      }
      frame "Update LED" {
        n117 = Variant To Data(error in=w371, type=T1 {"LED Indicator 1"=FALSE, "LED Indicator 2"=FALSE, "LED Indicator 3"=FALSE, "LED Indicator 4"=FALSE} ("LED Indicator"), Variant=w370) -> (data=w361:T1, error out=w366:errorcluster)
        n118 = Unbundle By Name(w373) -> ("FPGA Ref"=w369:refnum<k20>)
        n119 = call "Enqueue.vi"("Error In"=w366, "State"="IDLE", "Queue in"=w364) -> ("Error Out"=w365:errorcluster)  [unwired: 7 in, 1 out]
        n120 = Unbundle By Name(w361) -> ("LED Indicator 1"=w360:bool, "LED Indicator 2"=w359:bool, "LED Indicator 3"=w358:bool, "LED Indicator 4"=w357:bool)
        n121 = xnode "Read/Write Control"("FPGA VI Reference In"=w369, "error in"=w365, "Indicator LED-1"=w360, "Indicator LED-2"=w359, "Indicator LED-3"=w358, "Indicator LED-4"=w357) -> ("FPGA VI Reference Out"=w368:refnum<k20>, "error out"=w367:errorcluster)
        n122 = Bundle By Name(cluster=w373, "FPGA Ref"=w368) -> (w372:T4)
      }
      frame "IDLE" {
        (unwired) fxp<+,20,5> 0.0 ("SiPM data copy 1")
        n123 = Unbundle By Name(w416) -> ("FPGA Ref"=w415:refnum<k20>, "Mirror Change"=w411:enum16{"Camera Side", "SiPM Side"}, "Air Pressure Control.Air Compressor"=w398:bool, "Air Pressure Control.Air Compressor (Manual)"=w399:bool, "Air Pressure Control.Air Cmpressor Auto"=w397:bool)
        n124 = call "Enqueue.vi"("Error In"=w377, "State"="IDLE", "Queue in"=w375) -> ("Error Out"=w376:errorcluster)  [unwired: 7 in, 1 out]
        n125 = To Unsigned Byte Integer(number=w411) -> (unsigned 8bit integer=w408:u8)
        n126 = Select(t=w398, s=w399, f=w397) -> (s? t:f=w396:bool)
        n127 = Equal?(x=w408, y=u8 0) -> (x = y?=w407:bool)
        n128 = Equal?(x=w408, y=u8 1) -> (x = y?=w406:bool)
        n129 = call "TimerCounter.vi"("TriggerStatus"=w407) -> ("ResultOutput"=w405:bool)  [unwired: 9 in, 1 out]
        n130 = call "TimerCounter.vi"("TriggerStatus"=w406) -> ("ResultOutput"=w404:bool)  [unwired: 9 in, 1 out]
        n131 = xnode "Read/Write Control"("FPGA VI Reference In"=w415, "error in"=w376, "Mirror Change-A"=w405, "Mirror Change-B"=w404, "Air Compressor"=w396) -> ("FPGA VI Reference Out"=w413:refnum<k20>, "error out"=w393:errorcluster, "Lid Sensor-1"=w385:bool, "Lid Sensor-2"=w384:bool, "Lid Sensor-Laser Interlock"=w383:bool, "Level Sensor-3"=w382:bool, "Level Sensor-2"=w381:bool, "Level Sensor-1"=w380:bool, "SiPM data copy 1"=w379:fxp<+,20,5>, "SiPM data copy 2"=w378:fxp<+,20,5>, "Air Pressure Sensor"=w402:bool)
        n132 = Wait (ms)(milliseconds to wait=u32 100) -> ()  [unwired: 1 out]
        n133 = Not(x=w402) -> (.not. x?=w401:bool)
        n134 = call "TimerCounter.vi"("CounterTime(s)"=4.0, "TriggerStatus"=w402) -> ("ResultOutput"=w400:bool)  [unwired: 8 in, 1 out]
        n135 = Or(x=w401, y=w400) -> (x .or. y?=w395:bool)
        n136 = Bundle By Name(cluster=w416, "FPGA Ref"=w413, "Air Pressure Control.Air Cmpressor Auto"=w395) -> (w414:T4)
        n137 = To Double Precision Float(number=w379) -> (double precision float=→"SiPM 1":dbl)
        n138 = To Double Precision Float(number=w378) -> (double precision float=→"SiPM 2":dbl)
        n139 = Bundle By Name(cluster=T2 {"Lid Sensor 1"=FALSE, "Lid Sensor 2"=FALSE, "Laser Interlock"=FALSE, "Buffer Tank"=FALSE, "Wash Tank"=FALSE, "Waste Tank"=FALSE} ("Sensor Indicator"), "Lid Sensor 1"=w385, "Lid Sensor 2"=w384, "Laser Interlock"=w383, "Buffer Tank"=w382, "Wash Tank"=w381, "Waste Tank"=w380) -> (→"Sensor Indicator":T2)
        n140 = call "SEQ Preview Queue.vi"("error in"=w393) -> ("error out"=w394:errorcluster, "SEQ Data"=w391:T11)  [unwired: 9 in]
        n141 = Bundle By Name(cluster=w391, "Lid Sensor 1"=w385, "Lid Sensor 2"=w384, "Laser Interlock"=w383, "Buffer Tank"=w382, "Wash Tank"=w381, "Waste Tank"=w380, "SiPM 1"=w379, "SiPM 2"=w378) -> (w390:T11)
        n142 = call "SEQ Lossy Queue.vi"("error in"=w394, "SEQ Data"=w390) -> ("error out"=w392:errorcluster)  [unwired: 9 in]
      }
      frame "------Single Function------" {
      }
      frame "Buffer Load L" {
        w422 = T6 {"Wash Buffer Tank"=FALSE, "Buffer Load L"=FALSE, "Buffer Pump"=FALSE}  # Buffer Load L
        n143 = Unbundle By Name(w428) -> ("FPGA Ref"=w426:refnum<k20>)
        n144 = Variant To Data(error in=w430, type=w422, Variant=w429) -> (data=w423:T6, error out=w424:errorcluster)
        n145 = Unbundle By Name(w423) -> ("Wash Buffer Tank"=w421:bool, "Buffer Load L"=w420:bool, "Buffer Pump"=w419:bool)
        n146 = xnode "Read/Write Control"("FPGA VI Reference In"=w426, "Buffer Pinch Valve- 9"=w421, "Buffer Pinch Valve- 1"=w420, "Buffer Pump"=w419) -> ("FPGA VI Reference Out"=w425:refnum<k20>)  [unwired: 1 in, 1 out]
        n147 = Bundle By Name(cluster=w428, "FPGA Ref"=w425) -> (w427:T4)
      }
      frame "Buffer Load R" {
        w434 = T7 {"Wash Buffer Tank"=FALSE, "Buffer Load R"=FALSE, "Buffer Pump"=FALSE}  # Buffer Load R
        n148 = Unbundle By Name(w440) -> ("FPGA Ref"=w438:refnum<k20>)
        n149 = Variant To Data(error in=w442, type=w434, Variant=w441) -> (data=w435:T7, error out=w436:errorcluster)
        n150 = Unbundle By Name(w435) -> ("Wash Buffer Tank"=w433:bool, "Buffer Load R"=w432:bool, "Buffer Pump"=w431:bool)
        n151 = xnode "Read/Write Control"("FPGA VI Reference In"=w438, "Buffer Pinch Valve- 9"=w433, "Buffer Pinch Valve- 2"=w432, "Buffer Pump"=w431) -> ("FPGA VI Reference Out"=w437:refnum<k20>)  [unwired: 1 in, 1 out]
        n152 = Bundle By Name(cluster=w440, "FPGA Ref"=w437) -> (w439:T4)
      }
      frame "BL2" {
        w447 = cluster{"BL2":fxp<+,16,3>, "Buffer Chip L":bool} {"BL2"=0.0, "Buffer Chip L"=FALSE}  # BL2
        n153 = Unbundle By Name(w451) -> ("FPGA Ref"=w449:refnum<k20>)
        n154 = Variant To Data(error in=w453, type=w447, Variant=w452) -> (data=w445:cluster{"BL2":fxp<+,16,3>, "Buffer Chip L":bool}, error out=w446:errorcluster)
        n155 = Unbundle By Name(w445) -> ("BL2"=w444:fxp<+,16,3>, "Buffer Chip L"=w443:bool)
        n156 = xnode "Read/Write Control"("FPGA VI Reference In"=w449, "regulatorcontrol2 (V)"=w444, "Buffer Pinch Valve- 3"=w443) -> ("FPGA VI Reference Out"=w448:refnum<k20>)  [unwired: 1 in, 1 out]
        n157 = Bundle By Name(cluster=w451, "FPGA Ref"=w448) -> (w450:T4)
      }
      frame "BL1" {
        w458 = cluster{"BL1":fxp<+,16,3>, "Buffer Chip L":bool} {"BL1"=0.0, "Buffer Chip L"=FALSE}  # BL1
        n158 = Unbundle By Name(w462) -> ("FPGA Ref"=w460:refnum<k20>)
        n159 = Variant To Data(error in=w464, type=w458, Variant=w463) -> (data=w456:cluster{"BL1":fxp<+,16,3>, "Buffer Chip L":bool}, error out=w457:errorcluster)
        n160 = Unbundle By Name(w456) -> ("BL1"=w455:fxp<+,16,3>, "Buffer Chip L"=w454:bool)
        n161 = xnode "Read/Write Control"("FPGA VI Reference In"=w460, "regulatorcontrol1 (V)"=w455, "Buffer Pinch Valve- 3"=w454) -> ("FPGA VI Reference Out"=w459:refnum<k20>)  [unwired: 1 in, 1 out]
        n162 = Bundle By Name(cluster=w462, "FPGA Ref"=w459) -> (w461:T4)
      }
      frame "BR1" {
        w469 = cluster{"BR1":fxp<+,16,3>, "Buffer Chip R":bool} {"BR1"=0.0, "Buffer Chip R"=FALSE}  # BR1
        n163 = Unbundle By Name(w473) -> ("FPGA Ref"=w471:refnum<k20>)
        n164 = Variant To Data(error in=w475, type=w469, Variant=w474) -> (data=w467:cluster{"BR1":fxp<+,16,3>, "Buffer Chip R":bool}, error out=w468:errorcluster)
        n165 = Unbundle By Name(w467) -> ("BR1"=w466:fxp<+,16,3>, "Buffer Chip R"=w465:bool)
        n166 = xnode "Read/Write Control"("FPGA VI Reference In"=w471, "regulatorcontrol3 (V)"=w466, "Buffer Pinch Valve- 4"=w465) -> ("FPGA VI Reference Out"=w470:refnum<k20>)  [unwired: 1 in, 1 out]
        n167 = Bundle By Name(cluster=w473, "FPGA Ref"=w470) -> (w472:T4)
      }
      frame "BR2" {
        w480 = cluster{"BR2":fxp<+,16,3>, "Buffer Chip R":bool} {"BR2"=0.0, "Buffer Chip R"=FALSE}  # BR2
        n168 = Unbundle By Name(w484) -> ("FPGA Ref"=w482:refnum<k20>)
        n169 = Variant To Data(error in=w486, type=w480, Variant=w485) -> (data=w478:cluster{"BR2":fxp<+,16,3>, "Buffer Chip R":bool}, error out=w479:errorcluster)
        n170 = Unbundle By Name(w478) -> ("BR2"=w477:fxp<+,16,3>, "Buffer Chip R"=w476:bool)
        n171 = xnode "Read/Write Control"("FPGA VI Reference In"=w482, "regulatorcontrol4 (V)"=w477, "Buffer Pinch Valve- 4"=w476) -> ("FPGA VI Reference Out"=w481:refnum<k20>)  [unwired: 1 in, 1 out]
        n172 = Bundle By Name(cluster=w484, "FPGA Ref"=w481) -> (w483:T4)
      }
      frame "V1+BR1" {
        w492 = T8 {"BR1"=0.0, "Buffer Chip R"=FALSE, "Fast Valve 1"=FALSE}  # V1+BR1
        n173 = Unbundle By Name(w496) -> ("FPGA Ref"=w494:refnum<k20>)
        n174 = Variant To Data(error in=w498, type=w492, Variant=w497) -> (data=w490:T8, error out=w491:errorcluster)
        n175 = Unbundle By Name(w490) -> ("BR1"=w489:fxp<+,16,3>, "Buffer Chip R"=w488:bool, "Fast Valve 1"=w487:bool)
        n176 = xnode "Read/Write Control"("FPGA VI Reference In"=w494, "regulatorcontrol3 (V)"=w489, "Buffer Pinch Valve- 4"=w488, "FastValve1"=w487) -> ("FPGA VI Reference Out"=w493:refnum<k20>)  [unwired: 1 in, 1 out]
        n177 = Bundle By Name(cluster=w496, "FPGA Ref"=w493) -> (w495:T4)
      }
      frame "V2+BR2" {
        w504 = T9 {"BR2"=0.0, "Buffer Chip R"=FALSE, "Fast Valve 2"=FALSE}  # V2+BR2
        n178 = Unbundle By Name(w508) -> ("FPGA Ref"=w506:refnum<k20>)
        n179 = Variant To Data(error in=w510, type=w504, Variant=w509) -> (data=w502:T9, error out=w503:errorcluster)
        n180 = Unbundle By Name(w502) -> ("BR2"=w501:fxp<+,16,3>, "Buffer Chip R"=w500:bool, "Fast Valve 2"=w499:bool)
        n181 = xnode "Read/Write Control"("FPGA VI Reference In"=w506, "regulatorcontrol4 (V)"=w501, "Buffer Pinch Valve- 4"=w500, "FastValve2"=w499) -> ("FPGA VI Reference Out"=w505:refnum<k20>)  [unwired: 1 in, 1 out]
        n182 = Bundle By Name(cluster=w508, "FPGA Ref"=w505) -> (w507:T4)
      }
      frame "REA" {
        w515 = cluster{"BL2":fxp<+,16,3>, "Air Valve":bool} {"BL2"=0.0, "Air Valve"=FALSE}  # REA
        n183 = Unbundle By Name(w519) -> ("FPGA Ref"=w517:refnum<k20>)
        n184 = Variant To Data(error in=w521, type=w515, Variant=w520) -> (data=w513:cluster{"BL2":fxp<+,16,3>, "Air Valve":bool}, error out=w514:errorcluster)
        n185 = Unbundle By Name(w513) -> ("BL2"=w512:fxp<+,16,3>, "Air Valve"=w511:bool)
        n186 = xnode "Read/Write Control"("FPGA VI Reference In"=w517, "regulatorcontrol2 (V)"=w512, "Air Valve"=w511) -> ("FPGA VI Reference Out"=w516:refnum<k20>)  [unwired: 1 in, 1 out]
        n187 = Bundle By Name(cluster=w519, "FPGA Ref"=w516) -> (w518:T4)
      }
      frame "SW1/2" {
        w525 = cluster{"Sorting Waste":bool} {"Sorting Waste"=FALSE}  # SW1/2
        n188 = Unbundle By Name(w529) -> ("FPGA Ref"=w527:refnum<k20>)
        n189 = Variant To Data(error in=w531, type=w525, Variant=w530) -> (data=w523:cluster{"Sorting Waste":bool}, error out=w524:errorcluster)
        n190 = Unbundle By Name(w523) -> ("Sorting Waste"=w522:bool)
        n191 = xnode "Read/Write Control"("FPGA VI Reference In"=w527, "Buffer Pinch Valve- 5"=w522) -> ("FPGA VI Reference Out"=w526:refnum<k20>)  [unwired: 1 in, 1 out]
        n192 = Bundle By Name(cluster=w529, "FPGA Ref"=w526) -> (w528:T4)
      }
      frame "FW1/2" {
        w535 = cluster{"Filter Waste":bool} {"Filter Waste"=FALSE}  # FW1/2
        n193 = Unbundle By Name(w539) -> ("FPGA Ref"=w537:refnum<k20>)
        n194 = Variant To Data(error in=w541, type=w535, Variant=w540) -> (data=w533:cluster{"Filter Waste":bool}, error out=w534:errorcluster)
        n195 = Unbundle By Name(w533) -> ("Filter Waste"=w532:bool)
        n196 = xnode "Read/Write Control"("FPGA VI Reference In"=w537, "Buffer Pinch Valve- 6"=w532) -> ("FPGA VI Reference Out"=w536:refnum<k20>)  [unwired: 1 in, 1 out]
        n197 = Bundle By Name(cluster=w539, "FPGA Ref"=w536) -> (w538:T4)
      }
      frame "------Error Handler------" {
      }
      frame "Error" {
        n198 = Variant To Data(error in=w547, type=errorcluster {"status"=FALSE, "code"=0, "source"=""} ("error constant"), Variant=w546) -> (data=w548:errorcluster)  [unwired: 1 out]
        n199 = call <vilib>:"Simple Error Handler.vi"("error in (no error)"=w548) -> ()  [unwired: 4 in, 5 out]
      }
      frame "------Close------" {
      }
      frame "Close" {
        n200 = for {
          tunnel: w554 -> [w558]
          shift-right: [w559] -> w553
          shift-left: w555 -> [w560]
          tunnel: string[] ["Close Device", "Release Queue"] -> [w557] mode=indexing
          n201 = call "Enqueue.vi"("Error In"=w560, "State"=w557, "Queue in"=w558) -> ("Error Out"=w559:errorcluster)  [unwired: 7 in, 1 out]
        }
      }
      frame "Close Device" {
        n202 = Unbundle By Name(w563) -> ("FPGA Ref"=w562:refnum<k20>)
        n203 = xnode "Close FPGA VI Reference"("FPGA VI Reference In"=w562, "error in"=w564) -> ("error out"=w561:errorcluster)
      }
      frame "Release Queue" {
        n204 = Release Queue(queue=w568, error in (no error)=w569) -> (error out=w566:errorcluster)  [unwired: 1 in, 2 out]
        n205 = call "SEQ Release Queue.vi"("error in"=w566) -> ("error out"=w565:errorcluster)  [unwired: 10 in]
      }
    }
    n206 = case shown="Error .." w221 {
      selector: w221 -> [w571 w575]
      tunnel: [w571 w576] -> w222
      tunnel: w220 -> [_ w573]
      frame No Error {
      }
      frame Error {
        n207 = To Variant(anything=w575) -> (Variant=w574:variant)
        n208 = call "Enqueue.vi"("Data"=w574, "State"="Error", "Queue in"=w573) -> ("Error Out"=w576:errorcluster)  [unwired: 7 in, 1 out]
      }
    }
  }
  n209 = Merge Errors(w8, w6) -> (→"error out":errorcluster)
